vi "Set_RegGroup.vi"(8 "error in (no error)":errorcluster, 10 "data":T1, 11 "IB_RegGroup in":refnum<class "IB_RegGroup.lvclass">) -> (0 "error out":errorcluster, 3 "IB_RegGroup out":refnum<class "IB_RegGroup.lvclass">)   [LabVIEW 2020, in "IB_RegGroup.lvclass"]
uses:
  <vilib>/AppBuilder/IB_Classes/RegGroup/IB_RegGroup.lvclass
  <vilib>/AppBuilder/IB_Classes/RegGroup/IB_RegGroup.lvclass/IB_RegGroup.ctl
  <vilib>/AppBuilder/IB_Classes/RegData/IB_RegData.lvclass
  <vilib>/AppBuilder/IB_Classes/RegGroup/IB_RegGroup.ctl
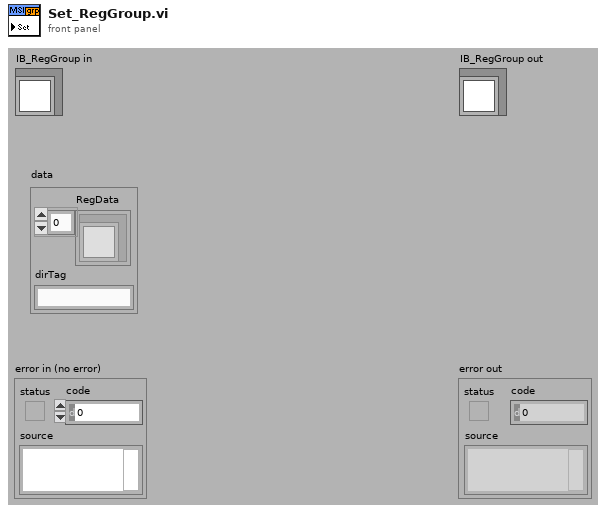
[diagram p1: front panel]
types:
  T1 = typedef "IB_RegGroup.ctl" = cluster{"RegData":refnum<class "IB_RegData.lvclass">[], "dirTag":string}
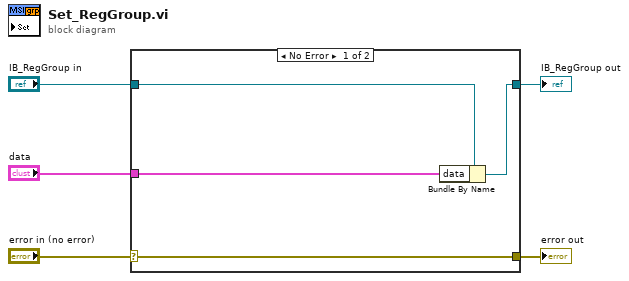
[diagram p0: block diagram]
diagram:
  n1 = case shown="No Error" "error in (no error)" {
    selector: "error in (no error)" -> [w9 w10]
    tunnel: [w9 w10] -> w4
    tunnel: [w7 w11] -> w2
    tunnel: "IB_RegGroup in" -> [w8 w11]
    tunnel: "data" -> [w6 _]
    frame No Error {
      n2 = Bundle By Name(cluster=w8, "data"=w6) -> (w7:refnum<class "IB_RegGroup.lvclass">)
    }
    frame Error {
    }
  }
  "error out" <- w4
  "IB_RegGroup out" <- w2
